vi "progress bar GV.vi"() -> ()   [LabVIEW 2017, in "util.lvlib"]
uses:
  util.lvlib
panel:
  in  "progress bar (ref)":refnum<vi>
  in  "progress bar text (ref)":refnum<vi>
  in  "value (0-100)":dbl format="%#_13g"
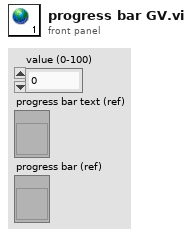
[diagram p1: front panel]
diagram:
